vi "phase to time.vi"(1 "data":cluster{"Array":dbl[], "Array":dbl[]}[](array[cluster])) -> (0 "data":cluster{"Array":dbl[], "Array":dbl[]}[](array[cluster]))   [LabVIEW 2021]
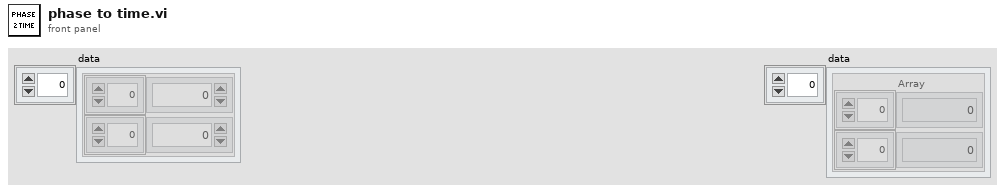
[diagram p1: front panel]
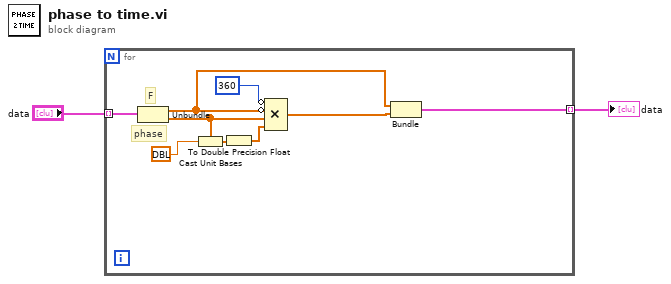
[diagram p0: block diagram]
diagram:
  n1 = for {
    tunnel: "data" -> [w11] mode=indexing
    tunnel: [w3] -> w1 mode=indexing
    # "phase"
    # "F"
    n2 = Unbundle(w11) -> ("Array"=w4:dbl[], "Array"=w8:dbl[])
    n3 = Cast Unit Bases(0:ext[unit] 299792458.0, 1:w8) -> (2:w7:ext[])
    n4 = To Double Precision Float(number=w7) -> (double precision float=w6:dbl[])
    n5 = Compound Arithmetic op=MULTIPLY(invert 360 ("frequncy"), invert w4, w8, w6) -> (w5:dbl[])
    n6 = Bundle("Array"=w4, w5) -> (w3:cluster{"Array":dbl[], dbl[]})  [unwired: 1 in]
  }
  "data" <- w1
